vi "ArrDevMeasAction.vi"(6 "Scan":bool, 7 "DevId":i32, 8 "error in (no error)":errorcluster caption="entrée d'erreur (pas d'erreur)", 9 "CurvePointIndex":i32, 10 "AllPointIndex":i32, 11 "Device In":refnum<class "ThorCCS200.lvclass"> caption="DNL_LabVIEW Object in") -> (0 "error out":errorcluster caption="sortie d'erreur", 1 "ArrDevDat":T1[](array[typedef]), 2 "ArrDevDatOut":dbl[][](array[numeric]), 3 "Device Out":refnum<class "ThorCCS200.lvclass"> caption="DNL_LabVIEW Object out", 5 "MeasOut":dbl[](array[numeric]))   [LabVIEW 2019, in "ThorCCS200.lvclass"]
uses:
  ThorCCS200.lvclass
  C:/Programmes Labview/LabscanV1A/DevicesClass/BaseDevice/BaseDevice.lvclass
  Experiment Class/ArrDevData.ctl
  ThorCCS200.lvclass/ThorCCS200.ctl
  <userlib>/GenProg/T_At_Wire/T_At_Wire_Err.vi
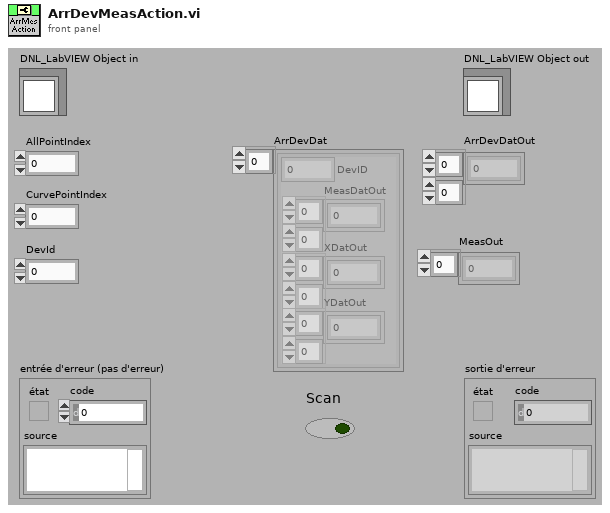
[diagram p1: front panel]
types:
  T1 = typedef "ArrDevData.ctl" = cluster{"MeasDatOut":dbl[][], "XDatOut":dbl[][], "YDatOut":dbl[][], "DevID":i32}
  T2 = typedef "ThorCCS200.lvclass/ThorCCS200_Func.ctl" = enum16{"ReadSpectrum (Acq)"}
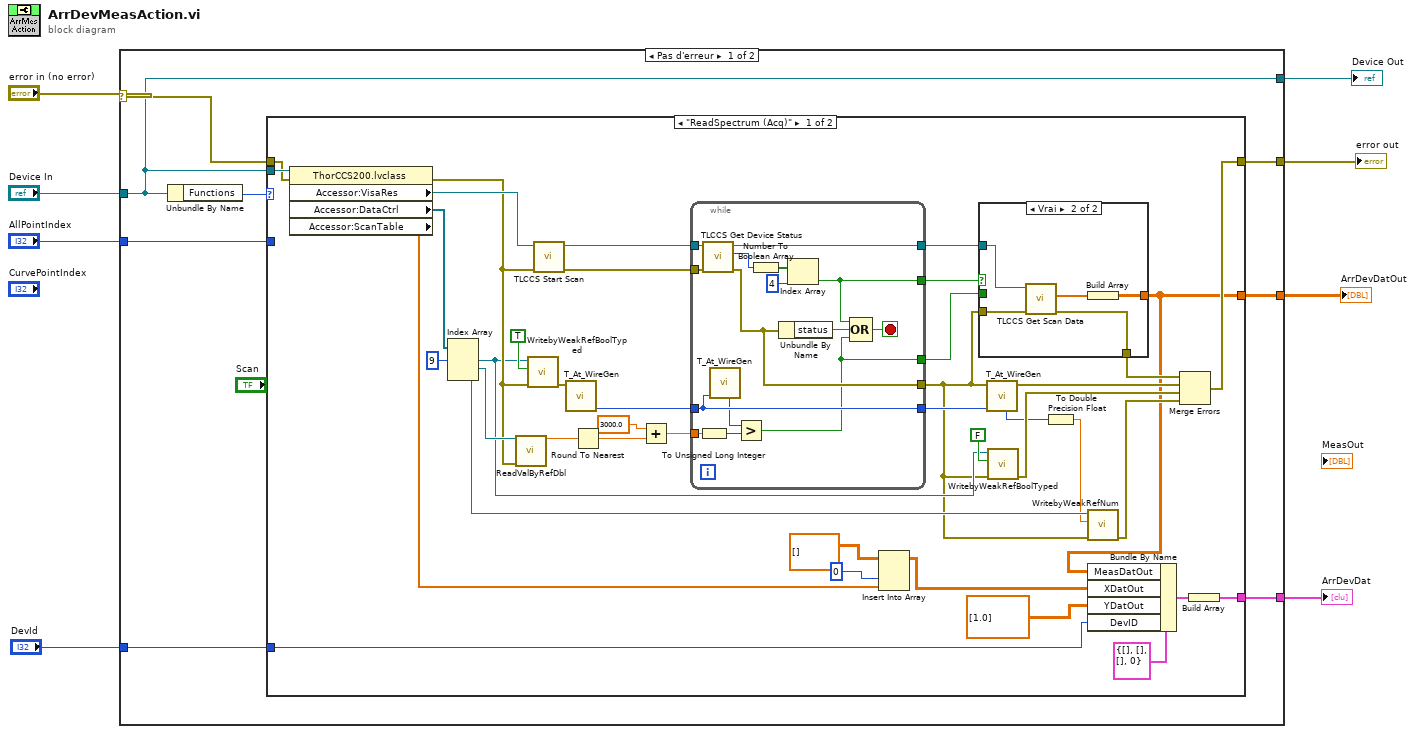
[diagram p0: block diagram]
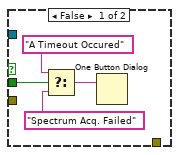
[diagram p2: hidden frame]
diagram:
  n1 = case shown="Pas d'erreur" "error in (no error)" {
    selector: "error in (no error)" -> [w14 w83]
    tunnel: "Device In" -> [w13 w84]
    tunnel: [w15 w83] -> w6
    tunnel: [w13 w84] -> w5
    tunnel: [w12 _] -> w4
    tunnel: [w11 _] -> w3
    tunnel: "DevId" -> [w10 _]
    tunnel: "AllPointIndex" -> [w9 _]
    frame No Error {
      n2 = Unbundle By Name(w13) -> ("Functions"=w16:T2)
      n3 = case shown="\"ReadSpectrum (Acq)\"" w16 {
        tunnel: [w34 w82] -> w15
        tunnel: w14 -> [w55 w82]
        tunnel: w13 -> [w57 _]
        tunnel: [w25 _] -> w12
        tunnel: [w24 _] -> w11
        tunnel: w10 -> [w18 _]
        tunnel: w9 -> [_ _]
        frame "ReadSpectrum (Acq)" {
          n4 = property class="ThorCCS200.lvclass"(reference=w57, error in=w55) -> (error out=w46:errorcluster, "Accessor:VisaRes"=w56:refnum<visa-resource-name>, "Accessor:DataCtrl"=w52:refnum<vi>[], "Accessor:ScanTable"=w20:dbl[])  [unwired: 1 out]
          n5 = Index Array(array=w52, index #1=9 ("indice")) -> (element #1=w38:refnum<vi>, element #2=w47:refnum<vi>, element #3=w32:refnum<vi>)  [unwired: 2 in]
          n6 = call <userlib>:"ReadValByRefDbl.vi"("Control Ref"=w47, "error in"=w46) -> ("Valeur"=w43:dbl)  [unwired: 12 in, 1 out]
          n7 = call <userlib>:"WritebyWeakRefBoolTyped.vi"("error in"=w46, "Valeur"=TRUE, "Control Ref"=w38) -> ("error out"=w50:errorcluster)  [unwired: 8 in]
          n8 = call <instrlib>:"TLCCS Start Scan.vi"("error in (no error)"=w46, "instrument handle"=w56) -> ("error out"=w54:errorcluster, "instrument handle out"=w53:refnum<visa-resource-name>)  [unwired: 8 in]
          n9 = call-poly <userlib>:"T_At_WireGen.vi"("error in (no error)"=w50) -> ("Clock(ms)"=w48:u32)  [unwired: 8 in, 2 out]
          n10 = Round To Nearest(number=w43) -> (nearest integer value=w45:dbl)
          n11 = Add(x=3000.0, y=w45) -> (x+y=w42:dbl)
          n12 = while {
            tunnel: w54 -> [w77]
            tunnel: w53 -> [w78]
            tunnel: [w76] -> w49
            tunnel: w48 -> [w76]
            tunnel: w42 -> [w71]
            tunnel: [w70] -> w29
            tunnel: [w69] -> w41
            tunnel: [w68] -> w40
            tunnel: [w67] -> w37
            stop <- w72 stop-if-true
            n13 = To Unsigned Long Integer(number=w71) -> (unsigned 32bit integer=w74:u32)
            n14 = call <instrlib>:"TLCCS Get Device Status.vi"("error in (no error)"=w77, "instrument handle"=w78) -> ("error out"=w70:errorcluster, "Device Status"=w81:i32, "instrument handle out"=w69:refnum<visa-resource-name>)  [unwired: 7 in]
            n15 = call-poly <userlib>:"T_At_WireGen.vi"("InitClock(ms)"=w76) -> ("Delta(ms)"=w75:u32)  [unwired: 8 in, 2 out]
            n16 = Greater?(x=w75, y=w74) -> (0:w67:bool)
            n17 = Number To Boolean Array(number=w81) -> (Boolean array=w80:bool[])
            n18 = Unbundle By Name(w70) -> ("status"=w73:bool)
            n19 = Index Array(array=w80, index=4) -> (element=w68:bool)
            n20 = Compound Arithmetic op=OR ("Opérateur arithmétique")(w68, w73, w67) -> (w72:bool)
          }
          n21 = Insert Into Array(array=dbl[][] [] ("tableau"), index (col)=0 ("indice désactivé (col)"), new element=w20) -> (w19:dbl[][])  [unwired: 1 in]
          n22 = case shown="Vrai" w40 {
            tunnel: w29 -> [_ w66]
            tunnel: [_ w64] -> w25
            tunnel: w41 -> [_ w63]
            tunnel: w37 -> [w61 _]
            tunnel: [_ w62] -> w33
            frame False {
              n23 = Select(t="A Timeout Occured", s=w61, f="Spectrum Acq. Failed") -> (s? t:f=w58:string)
              n24 = One Button Dialog(message=w58) -> ()  [unwired: 1 in, 1 out]
            }
            frame True {
              n25 = call <instrlib>:"TLCCS Get Scan Data.vi"("error in (no error)"=w66, "instrument handle"=w63) -> ("error out"=w62:errorcluster, "Data"=w65:dbl[])  [unwired: 7 in, 1 out]
              n26 = Build Array(w65) -> (w64:dbl[][])
            }
          }
          n27 = call-poly <userlib>:"T_At_WireGen.vi"("InitClock(ms)"=w49, "error in (no error)"=w29) -> ("error out"=w36:errorcluster, "Delta(ms)"=w31:u32)  [unwired: 7 in, 1 out]
          n28 = call <userlib>:"WritebyWeakRefBoolTyped.vi"("error in"=w29, "Valeur"=FALSE, "Control Ref"=w38) -> ("error out"=w35:errorcluster)  [unwired: 8 in]
          n29 = To Double Precision Float(number=w31) -> (double precision float=w30:dbl)
          n30 = call <userlib>:"WritebyWeakRefNum.vi"("error in"=w29, "Valeur"=w30, "Control Ref"=w32) -> ("error out"=w28:errorcluster)  [unwired: 8 in]
          n31 = Bundle By Name(cluster=T1 {"MeasDatOut"=[], "XDatOut"=[], "YDatOut"=[], "DevID"=0} ("cluster de sortie"), "MeasDatOut"=w25, "XDatOut"=w19, "YDatOut"=dbl[][] [[1.0]], "DevID"=w18) -> (w26:T1)
          n32 = Merge Errors(w33, w36, w35, w28) -> (w34:errorcluster)
          n33 = Build Array(w26) -> (w24:T1[])
        }
        frame Default {
        }
      }
    }
    frame Error {
    }
  }
  "error out" <- w6
  "Device Out" <- w5
  "ArrDevDatOut" <- w4
  "ArrDevDat" <- w3
